vi "ramp joystick.vi"(11 "joystick in":dbl) -> (3 "ramped joystick":dbl)   [LabVIEW 2011]
uses:
  <vilib>/addons/control/pid/pid.llb/PID (DBL).vi
  <vilib>/addons/control/pid/NI_PID_pid.lvlib
panel:
  out "dt out (s)":dbl format="%.3f"
  in  "PID gains":T1={"proportional gain (Kc)"=2.5, "integral time (Ti, min)"=0.0, "derivative time (Td, min)"=0.0} {"derivative time (Td, min)" format="%.3f"; "integral time (Ti, min)" format="%.3f"; "proportional gain (Kc)" format="%.3f"}
  out "Numeric":dbl
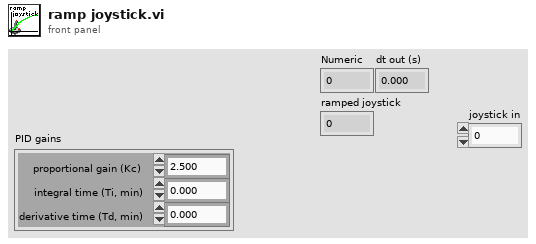
[diagram p1: front panel]
types:
  T1 = cluster{"proportional gain (Kc)":dbl, "integral time (Ti, min)":dbl, "derivative time (Td, min)":dbl}
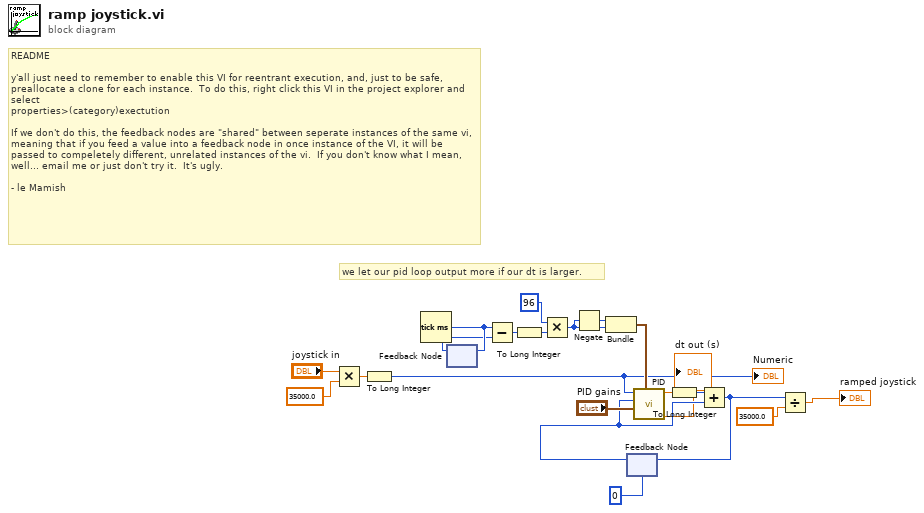
[diagram p0: block diagram]
diagram:
  # "README\n\ny'all just need to remember to enable this VI for reentrant execution, and, just to be safe, preallocate a clone for each instance.  To do this, right click this VI in the project explorer and select\nproperties>(category)exectution\n\nIf we don't do this, the feedback nodes are \"shared\" between seperate instances of the same vi, meaning that if you feed a value into a feedback node in once instance of the VI, it will be passed to compeletely different, unrelated instances of the vi.  If you don't know what I mean, well... email me or just don't try it.  It's ugly.\n\n- le Mamish"
  # "we let our pid loop output more if our dt is larger."
  n1 = Multiply(x="joystick in", y=35000.0) -> (x*y=w5:dbl)
  n2 = To Long Integer(number=w5) -> (32bit integer=w8:i32)
  "Numeric" <- w8
  n3 = Tick Count (ms)() -> (millisecond timer value=w16:u32)
  n4 = feedback #1() -> (w15:u32)  [unwired: 1 in]
  n5 = feedback-in #1(w16) -> ()
  n6 = Subtract(x=w16, y=w15) -> (x-y=w14:u32)
  n7 = To Long Integer(number=w14) -> (32bit integer=w12:i32)
  n8 = Multiply(x=96, y=w12) -> (x*y=w10:i32)
  n9 = Negate(x=w10) -> (-x=w11:i32)
  n10 = Bundle(w11, w10) -> (w9:cluster{i32, i32})  [unwired: 1 in]
  n11 = feedback #2(0) -> (w3:i32)
  n12 = call-poly <vilib>:"PID.vi"("output range"=w9, "PID gains"="PID gains", "process variable"=w3, "setpoint"=w8) -> ("dt out (s)"=→"dt out (s)":dbl, "output"=w19:dbl)  [unwired: 6 in]
  n13 = To Long Integer(number=w19) -> (32bit integer=w18:i32)
  n14 = Add(x=w18, y=w3) -> (x+y=w4:i32)
  n15 = feedback-in #2(w4) -> ()
  n16 = Divide(x=w4, y=35000.0) -> (x/y=→"ramped joystick":dbl)
